vi "Unregister Listener.vi"(8 "Error In":errorcluster, 11 "Listener ID":string) -> (0 "Error Out":errorcluster)   [LabVIEW 2025, in "LOGlib_LV2025.lvlib"]
doc: "Removes the listener from receiving logging statements."
uses:
  LOGlib_LV2025.lvlib
  Support/Action.ctl
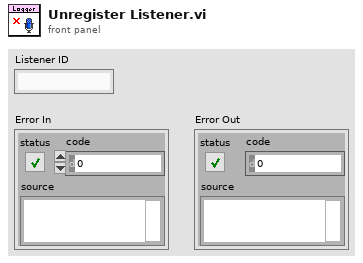
[diagram p1: front panel]
types:
  T1 = typedef "LOGlib_LV2025.lvlib/Action.ctl" = enum16{"Initialize", "Register", "Log", "Unregister", "Set Level", "Shutdown"}
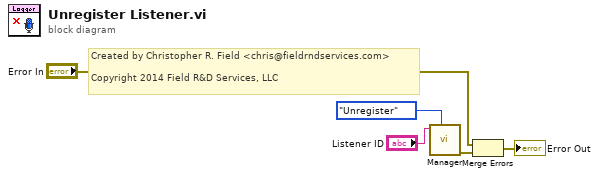
[diagram p0: block diagram]
diagram:
  # "Created by Christopher R. Field <chris@fieldrndservices.com>\n\nCopyright 2014 Field R&D Services, LLC"
  n1 = call "Manager.vi"("Action"=Action."Unregister", "Value In"="Listener ID") -> ("Error Out"=w3:errorcluster)  [unwired: 9 in]
  n2 = Merge Errors("Error In", w3) -> (→"Error Out":errorcluster)
